vi "AppMenuOptions.vi"(8 "error in (no error)":errorcluster, 10 "appMenu* in":refnum<k9>, 11 "xceRootNode in":refnum<class "xceRootNode.lvclass">) -> (0 "error out":errorcluster, 2 "appMenu* out":refnum<k9>, 3 "xceRootNode out":refnum<class "xceRootNode.lvclass">)   [LabVIEW 2013, in "xceRootNode.lvclass"]
uses:
  xceRootNode.lvclass
  <vilib>/Utility/miscctls.llb/LVMenuShortCut.ctl
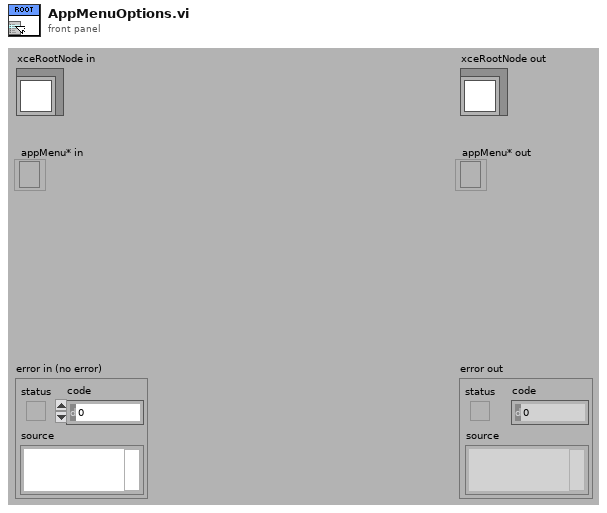
[diagram p1: front panel]
types:
  T1 = typedef "LVMenuShortCut.ctl" = cluster{"Include Shift Key?":bool, "Include Ctrl Key?":bool, "Shortcut Key":string}
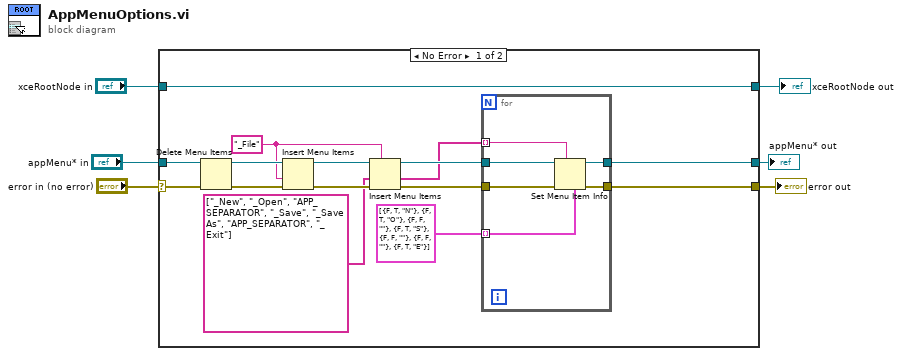
[diagram p0: block diagram]
diagram:
  n1 = case shown="No Error" "error in (no error)" {
    selector: "error in (no error)" -> [w17 w29]
    tunnel: [w8 w29] -> w5
    tunnel: [w21 w28] -> w3
    tunnel: "xceRootNode in" -> [w21 w28]
    tunnel: "appMenu* in" -> [w20 _]
    tunnel: [w7 _] -> w1
    frame No Error {
      w13 = "_File"
      n2 = Delete Menu Items(6:w17, 9:w20) -> (0:w18:errorcluster, 3:w19:refnum<k9>)  [unwired: 2 in]
      n3 = Insert Menu Items(6:w18, 7:w13, 9:w19) -> (0:w16:errorcluster, 3:w15:refnum<k9>)  [unwired: 3 in, 1 out]
      n4 = Insert Menu Items(5:w13, 6:w16, 7:string[] ["_New", "_Open", "APP_SEPARATOR", "_Save", "_Save As", "APP_SEPARATOR", "_Exit"], 9:w15) -> (0:w12:errorcluster, 1:w10:string[], 3:w11:refnum<k9>)  [unwired: 2 in]
      n5 = for {
        tunnel: w12 -> [w26]
        tunnel: w11 -> [w27]
        tunnel: w10 -> [w25] mode=indexing
        tunnel: T1[] [{"Include Shift Key?"=FALSE, "Include Ctrl Key?"=TRUE, "Shortcut Key"="N"}, {"Include Shift Key?"=FALSE, "Include Ctrl Key?"=TRUE, "Shortcut Key"="O"}, {"Include Shift Key?"=FALSE, "Include Ctrl Key?"=FALSE, "Shortcut Key"=""}, {"Include Shift Key?"=FALSE, "Include Ctrl Key?"=TRUE, "Shortcut Key"="S"}, {"Include Shift Key?"=FALSE, "Include Ctrl Key?"=FALSE, "Shortcut Key"=""}, {"Include Shift Key?"=FALSE, "Include Ctrl Key?"=FALSE, "Shortcut Key"=""}, {"Include Shift Key?"=FALSE, "Include Ctrl Key?"=TRUE, "Shortcut Key"="E"}] -> [w24] mode=indexing
        tunnel: [w23] -> w8
        tunnel: [w22] -> w7
        n6 = Set Menu Item Info(4:w24, 7:w25, 8:w26, 11:w27) -> (0:w23:errorcluster, 3:w22:refnum<k9>)  [unwired: 3 in]
      }
    }
    frame Error {
    }
  }
  "error out" <- w5
  "xceRootNode out" <- w3
  "appMenu* out" <- w1
